vi "Find Object Items by Name (Offset).vi"(7 "Item Names":string[](array[string]), 8 "error in (no error)":errorcluster, 10 "Object Offset (or Path)":i32, 11 "JSON":string) -> (0 "error out":errorcluster, 1 "<JSON>":string[](array[string]) caption="Items<JSON>", 2 "Found":bool[](array[boolean]))   [LabVIEW 2015, in "JSONtext.lvlib"]
uses:
  JSONtext.lvlib
  support/JSONtext support.lvlib
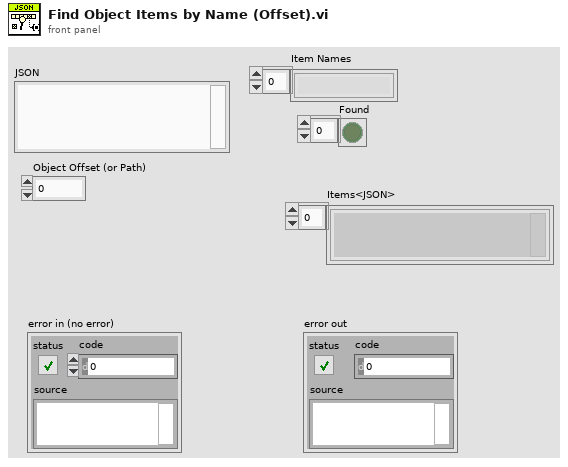
[diagram p1: front panel]
types:
  T1 = typedef "JSONtext.lvlib/Found Items.ctl" = cluster{"Item offset":i32, "Offset past Item":i32, "Name offset":i32, "Offset past Name":i32, "Found":bool, "Empty Object":bool}
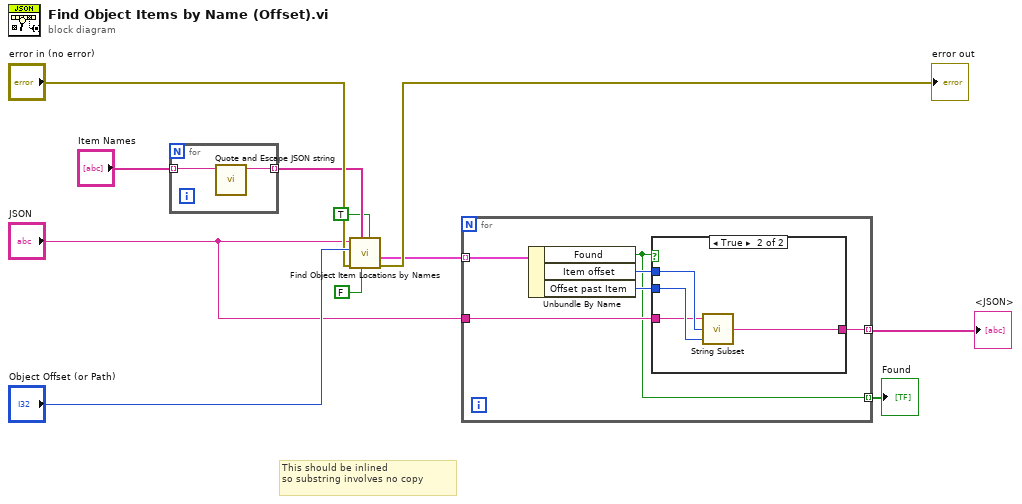
[diagram p0: block diagram]
diagram:
  # "This should be inlined\nso substring involves no copy"
  n1 = for {
    tunnel: "Item Names" -> [w13] mode=indexing
    tunnel: [w12] -> w3 mode=indexing
    n2 = call "Quote and Escape JSON string.vi"("Plain Text"=w13) -> ("<JSON>"=w12:string)  [unwired: 10 in]
  }
  n3 = call "Find Object Item Locations by Names.vi"("Insertion point if not found"=TRUE, "Only return first found"=FALSE, "Item Names <JSON>"=w3, "error in (no error)"="error in (no error)", "Object Offset"="Object Offset (or Path)", "JSON"="JSON") -> ("error out"=→"error out":errorcluster, "Items"=w6:T1[])  [unwired: 4 in]
  n4 = for {
    tunnel: "JSON" -> [w19]
    tunnel: [w18] -> w7 mode=indexing
    tunnel: w6 -> [w15] mode=indexing
    tunnel: [w14] -> w1 mode=indexing
    n5 = Unbundle By Name(w15) -> ("Found"=w14:bool, "Item offset"=w17:i32, "Offset past Item"=w16:i32)
    n6 = case shown="True" w14 {
      tunnel: w19 -> [_ w20]
      tunnel: [_ w23] -> w18
      tunnel: w17 -> [_ w22]
      tunnel: w16 -> [_ w21]
      frame False {
      }
      frame True {
        n7 = call "String Subset.vi"("Offset past End"=w21, "Start offset"=w22, "JSON"=w20) -> ("substring"=w23:string)  [unwired: 2 in]
      }
    }
  }
  "<JSON>" <- w7
  "Found" <- w1
